vi "Battery.vi"(8 "Battery Characterization":T1={"Battery Voltage"=12.9, "Internal Resistance"=0.015, "Battery Capacity"=64800.0, "Battery Temp"=75.0, "Battery Weight"=5.4431084400000005, "State of Charge %"=12.0} {"State of Charge %" format="%#_13g"; "Battery Weight" format="%#_13g"; "Battery Temp" format="%#_13g"; "Battery Capacity" format="%#_13g"; "Internal Resistance" format="%#_13g"; "Battery Voltage" format="%#_13g"}, 9 "Include Droop":bool=TRUE, 11 "Current":dbl[unit](slide) scale=0.0..1000.0) -> (2 "Battery Voltage":dbl[unit]=12.9 format="%#_13g")   [LabVIEW 2020]
uses:
  Battery Coefficients.ctl
  <vilib>/addons/control/pid/pid.llb/PID Control Input Filter (DBL).vi
  <vilib>/addons/control/pid/NI_PID_pid.lvlib
panel:
  out "Waveform Chart":cluster{dbl[unit], "Current":dbl[unit]}(graph)
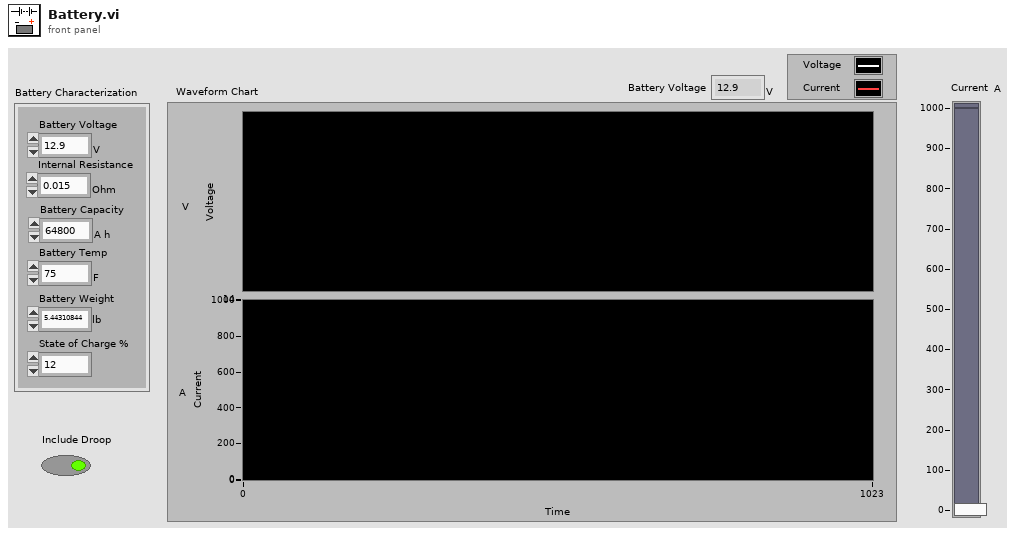
[diagram p1: front panel]
types:
  T1 = typedef "Battery Coefficients.ctl" = cluster{"Battery Voltage":dbl[unit], "Internal Resistance":dbl[unit], "Battery Capacity":dbl[unit], "Battery Temp":dbl[unit], "Battery Weight":dbl[unit], "State of Charge %":dbl}
  T2 = cluster{"Battery Voltage":dbl[unit], "Current":dbl[unit]}
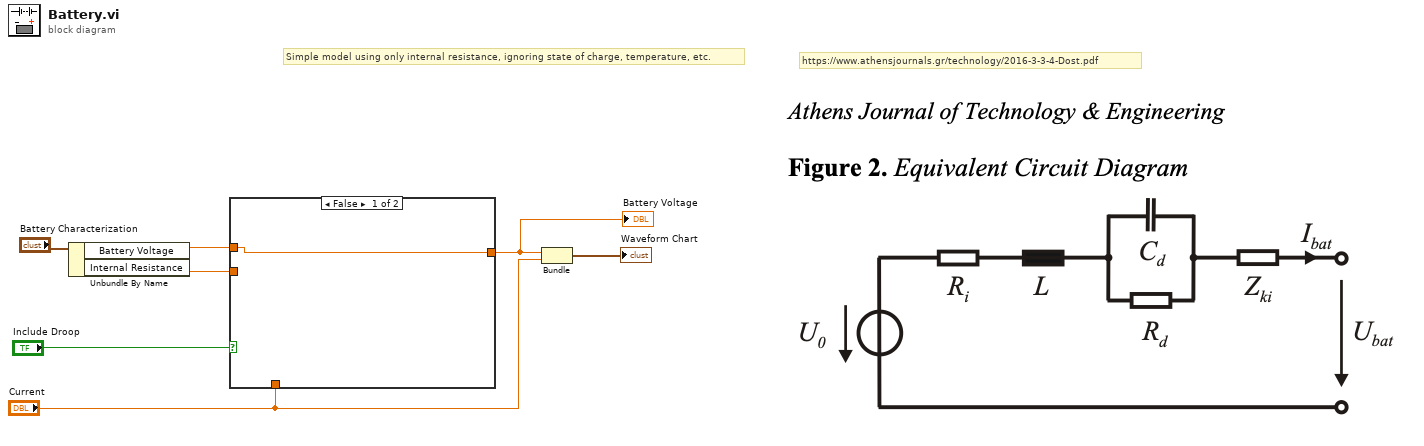
[diagram p0: block diagram]
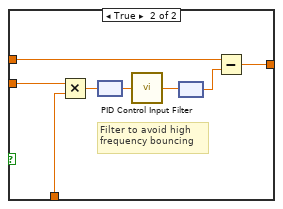
[diagram p2: hidden frame]
diagram:
  # "Simple model using only internal resistance, ignoring state of charge, temperature, etc."
  # "https://www.athensjournals.gr/technology/2016-3-3-4-Dost.pdf"
  n1 = Unbundle By Name("Battery Characterization") -> ("Battery Voltage"=w3:dbl[unit], "Internal Resistance"=w6:dbl[unit])
  n2 = case shown="False" "Include Droop" {
    tunnel: w6 -> [_ w16]
    tunnel: "Current" -> [_ w15]
    tunnel: w3 -> [w8 w10]
    tunnel: [w8 w9] -> w2
    frame False {
    }
    frame True {
      # "Filter to avoid high\nfrequency bouncing"
      n3 = Multiply(x=w16, y=w15) -> (x*y=w14:dbl[unit])
      n4 = node(w14) -> (w13:dbl)
      n5 = call-poly <vilib>:"PID Control Input Filter.vi"("input"=w13) -> ("output"=w12:dbl)  [unwired: 4 in]
      n6 = node(w12) -> (w11:dbl[unit])
      n7 = Subtract(x=w10, y=w11) -> (x-y=w9:dbl[unit])
    }
  }
  "Battery Voltage" <- w2
  n8 = Bundle("Battery Voltage"=w2, "Current"="Current") -> (→"Waveform Chart":T2)  [unwired: 1 in]
